vi "Call.vi"() -> ()   [LabVIEW 2020]
uses:
  Hardware A/Data.ctl
  Data.ctl
  Hardware A/Hardware A.lvlib
  Hardware B.lvlib
panel:
  out "error out":errorcluster caption="Fehler (Ausgang)"
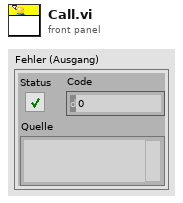
[diagram p1: front panel]
types:
  T1 = typedef "Hardware B.lvlib/Data.ctl" = cluster{"DeviceName":string}
  T2 = typedef "Hardware A.lvlib/Data.ctl" = cluster{"DeviceName":string}
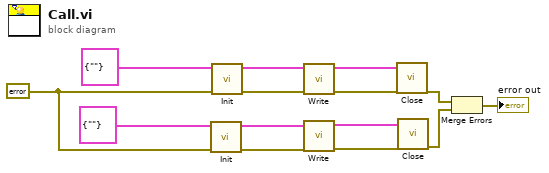
[diagram p0: block diagram]
diagram:
  w8 = errorcluster {"status"=FALSE, "code"=0, "source"=""} ("error out")
  n1 = call "Init.vi"("error in (no error)"=w8, "Data IN"=T1 {"DeviceName"=""}) -> ("error out"=w4:errorcluster, "Data Out"=w5:T1)  [unwired: 8 in]
  n2 = call "Init.vi"("error in (no error)"=w8, "Data IN"=T2 {"DeviceName"=""}) -> ("error out"=w13:errorcluster, "Data Out"=w14:T2)  [unwired: 8 in]
  n3 = call "Write.vi"("error in (no error)"=w13, "Data IN"=w14) -> ("error out"=w11:errorcluster, "Data IN"=w12:T2)  [unwired: 8 in]
  n4 = call "Write.vi"("error in (no error)"=w4, "Data IN"=w5) -> ("error out"=w2:errorcluster, "Data IN"=w3:T1)  [unwired: 8 in]
  n5 = call "Close.vi"("error in (no error)"=w11, "Data IN"=w12) -> ("error out"=w7:errorcluster)  [unwired: 8 in, 1 out]
  n6 = call "Close.vi"("error in (no error)"=w2, "Data IN"=w3) -> ("error out"=w1:errorcluster)  [unwired: 8 in, 1 out]
  n7 = Merge Errors(w7, w1) -> (→"error out":errorcluster)
